vi "GoTo.vi"(6 "Busy":refnum<vi>, 8 "error in (no error)":errorcluster, 10 "Param":string, 11 "Motor in":refnum<class "Motor.lvclass">) -> (0 "error out":errorcluster, 2 "Response":string, 3 "Motor out":refnum<class "Motor.lvclass">)   [LabVIEW 2012, in "Motor.lvclass"]
uses:
  Motor.lvclass
panel:
  out "VISA Mec":refnum<visa-resource-name>="COM6"
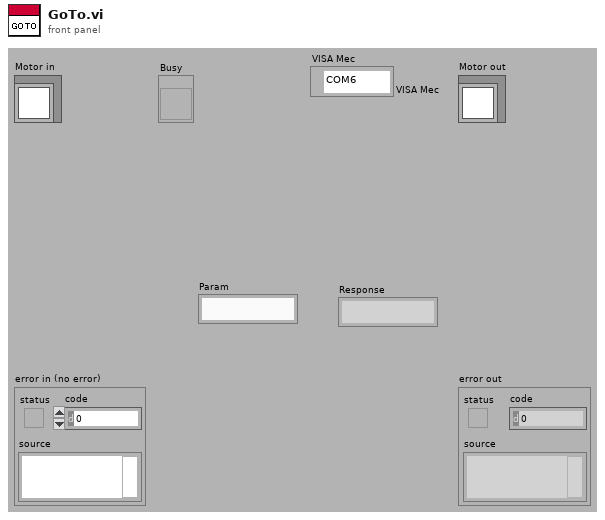
[diagram p1: front panel]
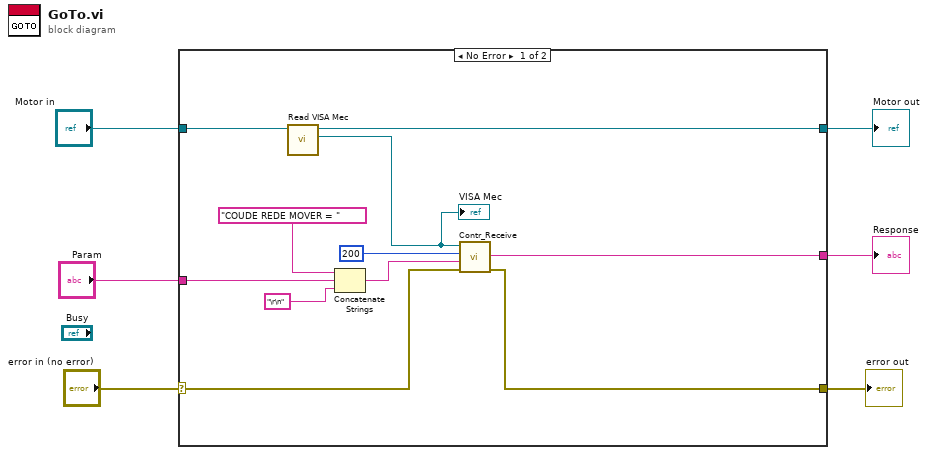
[diagram p0: block diagram]
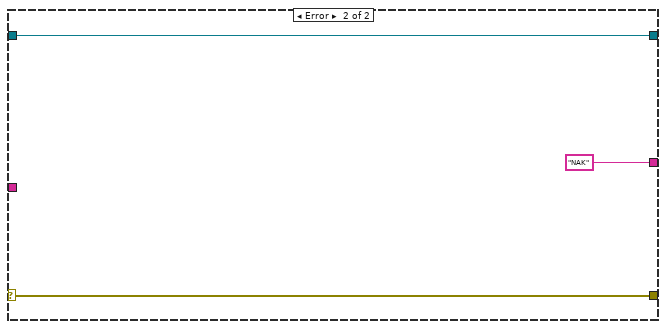
[diagram p2: hidden frame]
diagram:
  n1 = case shown="No Error" "error in (no error)" {
    selector: "error in (no error)" -> [w13 w19]
    tunnel: "Motor in" -> [w15 w20]
    tunnel: [w14 w20] -> w5
    tunnel: [w12 w19] -> w3
    tunnel: [w11 "NAK" ("Response from SIFS")] -> w2
    tunnel: "Param" -> [w9 _]
    frame No Error {
      n2 = call-dynamic "Read VISA Mec.vi"("Controlador in"=w15) -> ("VISA Mec"=w16:refnum<visa-resource-name>, "Controlador out"=w14:refnum<class "Motor.lvclass">)  [unwired: 8 in, 1 out]
      "VISA Mec" <- w16
      n3 = Concatenate Strings("COUDE REDE MOVER = " ("Command to SIFS"), w9, "\r\n" ("string")) -> (w7:string)
      n4 = call "Contr_Receive.vi"("error in"=w13, "Command to SIFS"=w7, "wait after tx"=u32 200, "VISA resource name"=w16) -> ("error out"=w12:errorcluster, "Response from SIFS"=w11:string)  [unwired: 2 out]
    }
    frame Error {
    }
  }
  "error out" <- w3
  "Motor out" <- w5
  "Response" <- w2
